vi "NiFpga_HdlFifo32_ReadBool.vi"(6 "timeout":u32, 7 "error in (no error)":errorcluster, 8 "number of elements":i32, 9 "fifo number":u32, 10 "fpga vi reference in":refnum<k20>) -> (0 "error out":errorcluster, 1 "elements remaining":u64, 2 "data out":bool[](array[boolean]), 3 "fpga vi reference out":refnum<k20>)   [LabVIEW 2023]
doc: "Dynamically reads the register at the provided offset. Set check for errors to true to check for errors such as if the register offset is invalid or if the register is running in an external clock domain that might not be running."
uses:
  NiFpga.dll
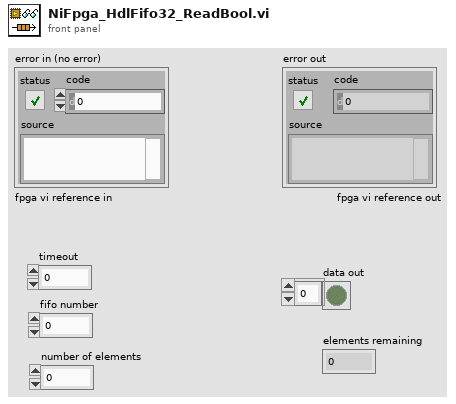
[diagram p1: front panel]
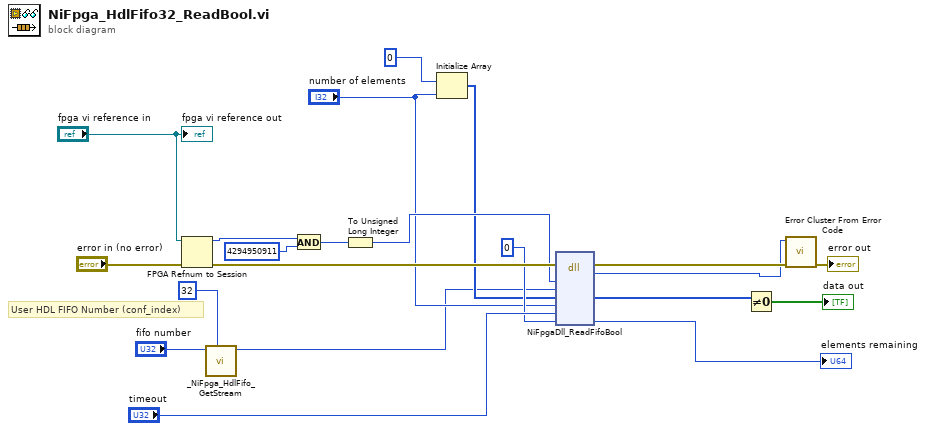
[diagram p0: block diagram]
diagram:
  # "User HDL FIFO Number (conf_index)"
  n1 = FPGA Refnum to Session(4:"error in (no error)", 7:"fpga vi reference in") -> (0:w16:errorcluster, 3:w18:u64)
  n2 = call "_NiFpga_HdlFifo_GetStream.vi"("NUM_DMA_CHANNELS"=u32 32, "Fifo Number"="fifo number") -> ("Fifo Stream"=w4:u32)  [unwired: 9 in]
  n3 = And(x=w18, y=u64 4294950911) -> (x .and. y?=w11:u64)
  n4 = To Unsigned Long Integer(number=w11) -> (unsigned 32bit integer=w10:u32)
  n5 = Initialize Array(u8 0, "number of elements") -> (w7:u8[])
  n6 = dll-call lib="NiFpga.*" fn="NiFpgaDll_ReadFifoBool"(error in=w16, "session"=w10, "fifo"=w4, "data"=w7, "numberOfElements"="number of elements", "timeout"="timeout", "elementsRemainining"=u64 0 ("emptyElementsRemainining")) -> (error out=w15:errorcluster, "return type"=w14:i32, "data"=w3:u8[], "elementsRemainining"=→"elements remaining":u64)  [unwired: 6 in, 1 out]
  n7 = Not Equal To 0?(x=w3) -> (x != 0?=→"data out":bool[])
  n8 = call <vilib>:"Error Cluster From Error Code.vi"("error in (no error)"=w15, "error code (0)"=w14) -> ("error out"=→"error out":errorcluster)  [unwired: 7 in]
  "fpga vi reference out" <- "fpga vi reference in"
